vi "MotorJudgePosition.vi"(3 "是否需要测量进度":bool, 4 "位置":dbl, 5 "直线电机？":bool, 6 "axis":i32) -> (1 "out":bool)   [LabVIEW 2018]
panel:
  out "通信成功？":bool
  out "初始化成功成功？":bool
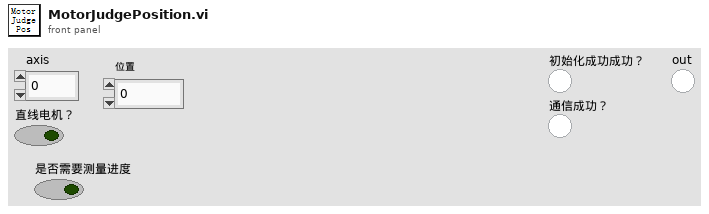
[diagram p1: front panel]
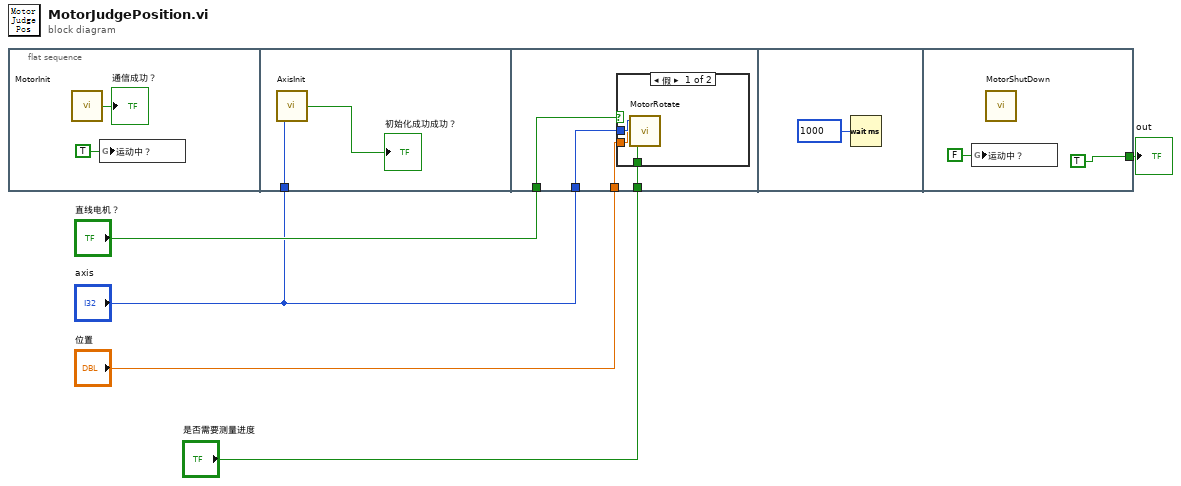
[diagram p0: block diagram]
diagram:
  n1 = flat-sequence {
    tunnel: "axis" -> [w9]
    tunnel: "axis" -> [w13]
    tunnel: "直线电机？" -> [w12]
    tunnel: "位置" -> [w11]
    tunnel: "是否需要测量进度" -> [w10]
    tunnel: [TRUE] -> w2
    frame #0 {
      n2 = call "MotorInit.vi"() -> ("通信成功？"=→"通信成功？":bool)  [unwired: 1 in]
      n3 = global write "globalMessage.vi" "运动中？"(TRUE ("运动中？")) -> ()
    }
    frame #1 {
      n4 = call "AxisInit.vi"("axis"=w9) -> ("初始化成功成功？"=→"初始化成功成功？":bool)
    }
    frame #2 {
      n5 = case shown="假" w12 {
        tunnel: w13 -> [w16 _]
        tunnel: w11 -> [w15 _]
        tunnel: w10 -> [w14 _]
        frame False {
          n6 = call "MotorRotate.vi"("是否需要测量进度？"=w14, "角度"=w15, "axis"=w16) -> ()  [unwired: 1 in, 1 out]
        }
        frame True {
        }
      }
    }
    frame #3 {
      n7 = Wait (ms)(milliseconds to wait=u32 1000 ("等待时间（毫秒）")) -> ()  [unwired: 1 out]
    }
    frame #4 {
      n8 = global write "globalMessage.vi" "运动中？"(FALSE ("运动中？")) -> ()
      n9 = call "MotorShutDown.vi"() -> ()  [unwired: 12 in]
    }
  }
  "out" <- w2
